vi "rs3 process filters.vi"(7 "Post-processing":T1, 8 "error in (no error)":errorcluster, 9 "Processing Queues":T3, 10 "Processing Blocks":T4, 11 "Frame":u64) -> (0 "error out":errorcluster, 2 "Processing times":T2, 3 "processed frame":u64)   [LabVIEW 2017, in "libRealSense3.lvlib"]
doc: "Applies post-processing filter to the depth stream in the following order:\n\n1. Subsampling\n2. Transform to disparity space\n3. Spatial filter\n4. Temporal filter\n5. Transform back to depth space"
uses:
  libRealSense3.lvlib
panel:
  # "RS3 Process Filters"
  # "(C) Intel Corp.,  AGJ"
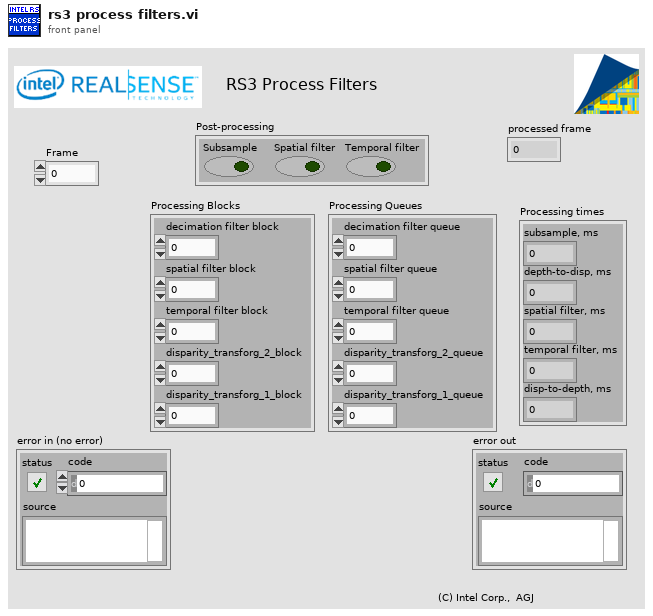
[diagram p1: front panel]
types:
  T1 = cluster{"Subsample":bool, "Spatial filter":bool, "Temporal filter":bool}
  T2 = cluster{"subsample, ms":u32, "depth-to-disp, ms":u32, "spatial filter, ms":u32, "temporal filter, ms":u32, "disp-to-depth, ms":u32}
  T3 = cluster{"decimation filter queue":u64, "spatial filter queue":u64, "temporal filter queue":u64, "disparity_transforg_2_queue":u64, "disparity_transforg_1_queue":u64}
  T4 = cluster{"decimation filter block":u64, "spatial filter block":u64, "temporal filter block":u64, "disparity_transforg_2_block":u64, "disparity_transforg_1_block":u64}
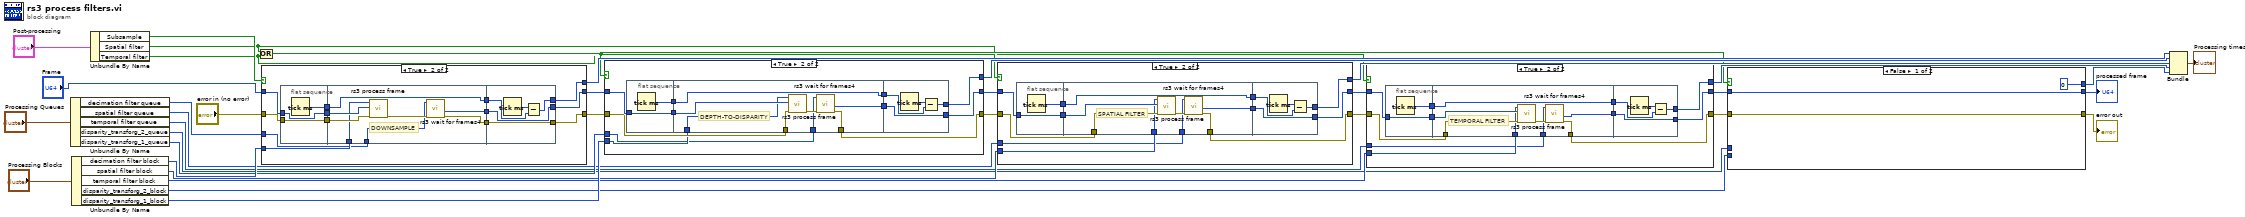
[diagram p0: block diagram]
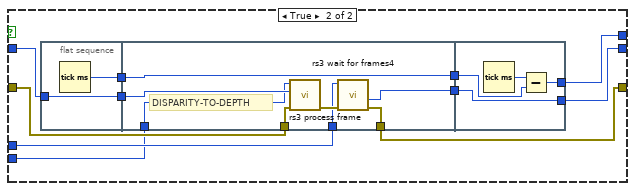
[diagram p2: hidden frame]
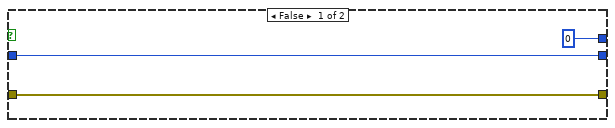
[diagram p3: hidden frame]
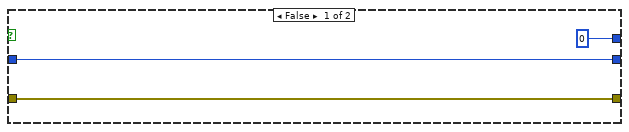
[diagram p4: hidden frame]
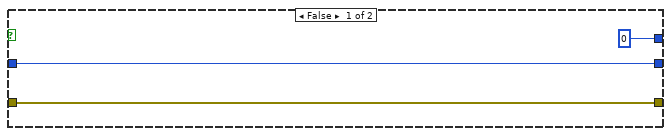
[diagram p5: hidden frame]
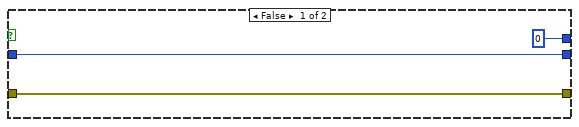
[diagram p6: hidden frame]
diagram:
  n1 = Unbundle By Name("Processing Queues") -> ("decimation filter queue"=w30:u64, "spatial filter queue"=w17:u64, "temporal filter queue"=w15:u64, "disparity_transforg_2_queue"=w14:u64, "disparity_transforg_1_queue"=w19:u64)
  n2 = Unbundle By Name("Processing Blocks") -> ("decimation filter block"=w31:u64, "spatial filter block"=w18:u64, "temporal filter block"=w16:u64, "disparity_transforg_2_block"=w13:u64, "disparity_transforg_1_block"=w20:u64)
  n3 = Unbundle By Name("Post-processing") -> ("Subsample"=w3:bool, "Spatial filter"=w2:bool, "Temporal filter"=w1:bool)
  n4 = Or(x=w2, y=w1) -> (x .or. y?=w6:bool)
  n5 = case shown="True" w3 {
    tunnel: "error in (no error)" -> [w37 w45]
    tunnel: "Frame" -> [w36 w44]
    tunnel: w31 -> [_ w43]
    tunnel: w30 -> [_ w42]
    tunnel: [w36 w41] -> w29
    tunnel: [w37 w40] -> w24
    tunnel: [u32 0 w39] -> w12
    frame False {
    }
    frame True {
      n6 = flat-sequence {
        tunnel: w44 -> [w53]
        tunnel: w45 -> [w54]
        tunnel: [w54] -> w51
        tunnel: [w53] -> w50
        tunnel: [w52] -> w49
        tunnel: w43 -> [w60]
        tunnel: w42 -> [w56]
        tunnel: w51 -> [w62]
        tunnel: w50 -> [w61]
        tunnel: [w58] -> w48
        tunnel: w49 -> [w58]
        tunnel: [w55] -> w47
        tunnel: [w57] -> w46
        tunnel: [w65] -> w41
        tunnel: w48 -> [w66]
        tunnel: w47 -> [w65]
        tunnel: [w64] -> w40
        tunnel: w46 -> [w64]
        tunnel: [w63] -> w39
        frame #0 {
          n7 = Tick Count (ms)() -> (millisecond timer value=w52:u32)
        }
        frame #1 {
          # "DOWNSAMPLE"
          n8 = call "rs3 process frame.vi"("error in (no error)"=w62, "Frame"=w61, "Processing Block"=w60) -> ("error out"=w59:errorcluster)  [unwired: 6 in, 2 out]
          n9 = call "rs3 wait for frames4.vi"("error in (no error)"=w59, "Queue in"=w56) -> ("error out"=w57:errorcluster, "frame"=w55:u64)  [unwired: 6 in, 2 out]
        }
        frame #2 {
          n10 = Tick Count (ms)() -> (millisecond timer value=w67:u32)
          n11 = Subtract(x=w67, y=w66) -> (x-y=w63:u32)
        }
      }
    }
  }
  n12 = case shown="True" w6 {
    tunnel: w29 -> [w69 w77]
    tunnel: [w69 w76] -> w28
    tunnel: w24 -> [w68 w75]
    tunnel: [w68 w74] -> w23
    tunnel: w20 -> [_ w73]
    tunnel: w19 -> [_ w72]
    tunnel: [u32 0 w71] -> w11
    frame False {
    }
    frame True {
      n13 = flat-sequence {
        tunnel: w77 -> [w83]
        tunnel: [w83] -> w81
        tunnel: [w82] -> w80
        tunnel: w81 -> [w91]
        tunnel: [w89] -> w79
        tunnel: w80 -> [w89]
        tunnel: [w84] -> w78
        tunnel: w75 -> [w88]
        tunnel: [w87] -> w74
        tunnel: w73 -> [w86]
        tunnel: w72 -> [w85]
        tunnel: [w93] -> w76
        tunnel: w79 -> [w94]
        tunnel: w78 -> [w93]
        tunnel: [w92] -> w71
        frame #0 {
          n14 = Tick Count (ms)() -> (millisecond timer value=w82:u32)
        }
        frame #1 {
          # "DEPTH-TO-DISPARITY"
          n15 = call "rs3 process frame.vi"("error in (no error)"=w88, "Frame"=w91, "Processing Block"=w86) -> ("error out"=w90:errorcluster)  [unwired: 6 in, 2 out]
          n16 = call "rs3 wait for frames4.vi"("error in (no error)"=w90, "Queue in"=w85) -> ("error out"=w87:errorcluster, "frame"=w84:u64)  [unwired: 6 in, 2 out]
        }
        frame #2 {
          n17 = Tick Count (ms)() -> (millisecond timer value=w95:u32)
          n18 = Subtract(x=w95, y=w94) -> (x-y=w92:u32)
        }
      }
    }
  }
  n19 = case shown="True" w2 {
    tunnel: w28 -> [w97 w105]
    tunnel: [w97 w104] -> w27
    tunnel: w23 -> [w96 w103]
    tunnel: [w96 w102] -> w22
    tunnel: w18 -> [_ w101]
    tunnel: w17 -> [_ w100]
    tunnel: [u32 0 w99] -> w10
    frame False {
    }
    frame True {
      n20 = flat-sequence {
        tunnel: w105 -> [w111]
        tunnel: [w111] -> w109
        tunnel: [w110] -> w108
        tunnel: w109 -> [w119]
        tunnel: [w117] -> w107
        tunnel: w108 -> [w117]
        tunnel: [w112] -> w106
        tunnel: w103 -> [w116]
        tunnel: [w115] -> w102
        tunnel: w101 -> [w113]
        tunnel: w100 -> [w114]
        tunnel: w107 -> [w122]
        tunnel: w106 -> [w121]
        tunnel: [w121] -> w104
        tunnel: [w120] -> w99
        frame #0 {
          n21 = Tick Count (ms)() -> (millisecond timer value=w110:u32)
        }
        frame #1 {
          # "SPATIAL FILTER"
          n22 = call "rs3 process frame.vi"("error in (no error)"=w116, "Frame"=w119, "Processing Block"=w113) -> ("error out"=w118:errorcluster)  [unwired: 6 in, 2 out]
          n23 = call "rs3 wait for frames4.vi"("error in (no error)"=w118, "Queue in"=w114) -> ("error out"=w115:errorcluster, "frame"=w112:u64)  [unwired: 6 in, 2 out]
        }
        frame #2 {
          n24 = Tick Count (ms)() -> (millisecond timer value=w123:u32)
          n25 = Subtract(x=w123, y=w122) -> (x-y=w120:u32)
        }
      }
    }
  }
  n26 = case shown="True" w1 {
    tunnel: w27 -> [w125 w133]
    tunnel: [w125 w132] -> w26
    tunnel: w22 -> [w124 w131]
    tunnel: [w124 w130] -> w21
    tunnel: w16 -> [_ w129]
    tunnel: w15 -> [_ w128]
    tunnel: [u32 0 w127] -> w9
    frame False {
    }
    frame True {
      n27 = flat-sequence {
        tunnel: w133 -> [w139]
        tunnel: [w139] -> w137
        tunnel: [w138] -> w136
        tunnel: w137 -> [w147]
        tunnel: [w145] -> w135
        tunnel: w136 -> [w145]
        tunnel: [w140] -> w134
        tunnel: w131 -> [w144]
        tunnel: [w143] -> w130
        tunnel: w129 -> [w142]
        tunnel: w128 -> [w141]
        tunnel: [w149] -> w132
        tunnel: w135 -> [w150]
        tunnel: w134 -> [w149]
        tunnel: [w148] -> w127
        frame #0 {
          n28 = Tick Count (ms)() -> (millisecond timer value=w138:u32)
        }
        frame #1 {
          # "TEMPORAL FILTER"
          n29 = call "rs3 process frame.vi"("error in (no error)"=w144, "Frame"=w147, "Processing Block"=w142) -> ("error out"=w146:errorcluster)  [unwired: 6 in, 2 out]
          n30 = call "rs3 wait for frames4.vi"("error in (no error)"=w146, "Queue in"=w141) -> ("error out"=w143:errorcluster, "frame"=w140:u64)  [unwired: 6 in, 2 out]
        }
        frame #2 {
          n31 = Tick Count (ms)() -> (millisecond timer value=w151:u32)
          n32 = Subtract(x=w151, y=w150) -> (x-y=w148:u32)
        }
      }
    }
  }
  n33 = case shown="False" w6 {
    tunnel: w26 -> [w153 w161]
    tunnel: [w153 w160] -> w25
    tunnel: w21 -> [w152 w159]
    tunnel: w14 -> [_ w158]
    tunnel: w13 -> [_ w157]
    tunnel: [u32 0 w156] -> w8
    tunnel: [w152 w155] -> w5
    frame False {
    }
    frame True {
      n34 = flat-sequence {
        tunnel: w161 -> [w167]
        tunnel: [w167] -> w165
        tunnel: [w166] -> w164
        tunnel: w165 -> [w175]
        tunnel: [w173] -> w163
        tunnel: w164 -> [w173]
        tunnel: [w168] -> w162
        tunnel: w159 -> [w172]
        tunnel: w158 -> [w169]
        tunnel: w157 -> [w171]
        tunnel: [w170] -> w155
        tunnel: [w177] -> w160
        tunnel: w163 -> [w178]
        tunnel: w162 -> [w177]
        tunnel: [w176] -> w156
        frame #0 {
          n35 = Tick Count (ms)() -> (millisecond timer value=w166:u32)
        }
        frame #1 {
          # "DISPARITY-TO-DEPTH"
          n36 = call "rs3 process frame.vi"("error in (no error)"=w172, "Frame"=w175, "Processing Block"=w171) -> ("error out"=w174:errorcluster)  [unwired: 6 in, 2 out]
          n37 = call "rs3 wait for frames4.vi"("error in (no error)"=w174, "Queue in"=w169) -> ("error out"=w170:errorcluster, "frame"=w168:u64)  [unwired: 6 in, 2 out]
        }
        frame #2 {
          n38 = Tick Count (ms)() -> (millisecond timer value=w179:u32)
          n39 = Subtract(x=w179, y=w178) -> (x-y=w176:u32)
        }
      }
    }
  }
  "processed frame" <- w25
  "error out" <- w5
  n40 = Bundle(w12, w11, w10, w9, w8) -> (→"Processing times":cluster{u32, u32, u32, u32, u32})  [unwired: 1 in]
